vi "median and quartiles.vi"(11 "Data":dbl[](array[numeric]) format="%#.6g") -> (1 "Lower quartile (LQ)":dbl format="%#.6g", 2 "Median":dbl format="%#.6g", 3 "Upper quartile (UQ)":dbl format="%#.6g")   [LabVIEW 2023]
doc: "Computes the median and upper and lower quartiles for the boxplot."
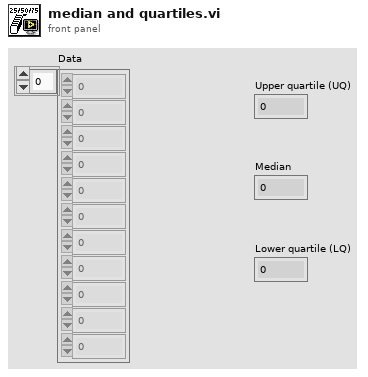
[diagram p1: front panel]
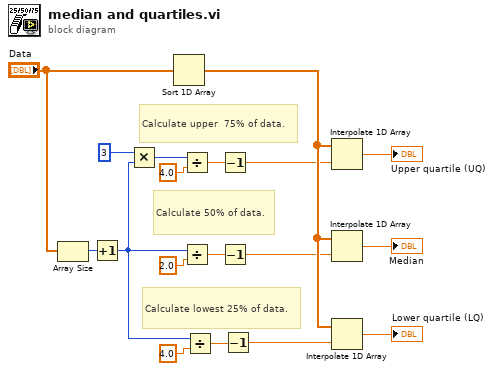
[diagram p0: block diagram]
diagram:
  # "Calculate 50% of data."
  # "Calculate lowest 25% of data."
  # "Calculate upper  75% of data."
  n1 = Array Size(array="Data") -> (size(s)=w2:i32)
  n2 = Increment(x=w2) -> (x+1=w1:i32)
  n3 = Multiply(x=3, y=w1) -> (x*y=w3:i32)
  n4 = Sort 1D Array(array="Data") -> (sorted array=w12:dbl[])
  n5 = Divide(x=w3, y=4.0) -> (x/y=w4:dbl)
  n6 = Divide(x=w1, y=2.0) -> (x/y=w9:dbl)
  n7 = Divide(x=w1, y=4.0) -> (x/y=w8:dbl)
  n8 = Decrement(x=w4) -> (x-1=w5:dbl)
  n9 = Decrement(x=w9) -> (x-1=w6:dbl)
  n10 = Decrement(x=w8) -> (x-1=w7:dbl)
  n11 = Interpolate 1D Array(1:w5, 2:w12) -> (0:→"Upper quartile (UQ)":dbl)
  n12 = Interpolate 1D Array(1:w6, 2:w12) -> (0:→"Median":dbl)
  n13 = Interpolate 1D Array(1:w7, 2:w12) -> (0:→"Lower quartile (LQ)":dbl)
